vi "Tx to UDP.vi"(7 "Data Conversion":T1, 8 "error in (no error)":errorcluster, 10 "Tx Array":dbl[](array[numeric]), 11 "Header Info":bool[](array[boolean])) -> (0 "error out":errorcluster, 2 "Tx String":string, 5 "Data Conversion out":T1)   [LabVIEW 2016, in "UDP-Custom-Device Engine.lvlib"]
uses:
  UDP-Custom-Device Engine.lvlib
  Types/Engine - Data Conversion Config.ctl
  <vilib>/NI Veristand/VeriStand Data/Library/Byte Buffer/Byte Buffer.lvclass
  <vilib>/NI Veristand/VeriStand Data/Library/Byte Buffer/Byte Buffer.Mapping.ctl
  <vilib>/NI Veristand/VeriStand Data/Library/Typedefs/Typedefs.Data Types.ctl
  <vilib>/NI Veristand/VeriStand Data/Library/Byte Buffer/Byte Buffer.lvclass/Byte Buffer.ctl
  <vilib>/NI Veristand/VeriStand Data/Library/Pointer Operations/Pointer.Write (DBL).vi
  <vilib>/NI Veristand/VeriStand Data/Library/Memory Management/Memory Management.MoveDblBlock.Write (Double).vi
  <vilib>/NI Veristand/VeriStand Data/Library/Byte Buffer/Byte Buffer.Write.Typed Array.vi
  <vilib>/NI Veristand/VeriStand Data/Library/Utilities/Utilities.Buffer.Double.vi
  <vilib>/NI Veristand/VeriStand Data/Library/Byte Buffer/Byte Buffer.Write.vi
  <vilib>/NI Veristand/VeriStand Data/Library/Byte Buffer/Byte Buffer.Write (1D Boolean).vi
  <vilib>/NI Veristand/VeriStand Data/Library/Type Conversion/Type Conversion.From Double.Subset.vi
  <vilib>/NI Veristand/VeriStand Data/Library/Type Conversion/Type Conversion.From Double.Subset (1D Boolean).vi
  <vilib>/NI Veristand/VeriStand Data/Library/Byte Buffer/Byte Buffer.Write (1D SGL).vi
  <vilib>/NI Veristand/VeriStand Data/Library/Type Conversion/Type Conversion.From Double.Subset (1D SGL).vi
  <vilib>/NI Veristand/VeriStand Data/Library/Byte Buffer/Byte Buffer.Write (1D DBL).vi
  <vilib>/NI Veristand/VeriStand Data/Library/Byte Buffer/Byte Buffer.Write (1D I8).vi
  <vilib>/NI Veristand/VeriStand Data/Library/Type Conversion/Type Conversion.From Double.Subset (1D I8).vi
  <vilib>/NI Veristand/VeriStand Data/Library/Byte Buffer/Byte Buffer.Write (1D I16).vi
  <vilib>/NI Veristand/VeriStand Data/Library/Type Conversion/Type Conversion.From Double.Subset (1D I16).vi
  <vilib>/NI Veristand/VeriStand Data/Library/Byte Buffer/Byte Buffer.Write (1D I32).vi
  <vilib>/NI Veristand/VeriStand Data/Library/Type Conversion/Type Conversion.From Double.Subset (1D I32).vi
  <vilib>/NI Veristand/VeriStand Data/Library/Byte Buffer/Byte Buffer.Write (1D I64).vi
  <vilib>/NI Veristand/VeriStand Data/Library/Type Conversion/Type Conversion.From Double.Subset (1D I64).vi
  <vilib>/NI Veristand/VeriStand Data/Library/Byte Buffer/Byte Buffer.Write (1D U8).vi
  <vilib>/NI Veristand/VeriStand Data/Library/Type Conversion/Type Conversion.From Double.Subset (1D U8).vi
  <vilib>/NI Veristand/VeriStand Data/Library/Byte Buffer/Byte Buffer.Write (1D U16).vi
  <vilib>/NI Veristand/VeriStand Data/Library/Type Conversion/Type Conversion.From Double.Subset (1D U16).vi
  <vilib>/NI Veristand/VeriStand Data/Library/Byte Buffer/Byte Buffer.Write (1D U32).vi
  <vilib>/NI Veristand/VeriStand Data/Library/Type Conversion/Type Conversion.From Double.Subset (1D U32).vi
  <vilib>/NI Veristand/VeriStand Data/Library/Byte Buffer/Byte Buffer.Write (1D U64).vi
  <vilib>/NI Veristand/VeriStand Data/Library/Type Conversion/Type Conversion.From Double.Subset (1D U64).vi
  <vilib>/NI Veristand/VeriStand Data/Library/Utilities/Utilities.Sizeof.Array.vi
  <vilib>/NI Veristand/VeriStand Data/Library/Type Conversion/Type Conversion.From Double.vi
  <vilib>/NI Veristand/VeriStand Data/Library/Type Conversion/Type Conversion.From Double (1D Boolean).vi
  <vilib>/NI Veristand/VeriStand Data/Library/Type Conversion/Type Conversion.From Double (1D SGL).vi
  <vilib>/NI Veristand/VeriStand Data/Library/Type Conversion/Type Conversion.From Double (1D I8).vi
  <vilib>/NI Veristand/VeriStand Data/Library/Type Conversion/Type Conversion.From Double (1D I16).vi
  <vilib>/NI Veristand/VeriStand Data/Library/Type Conversion/Type Conversion.From Double (1D I32).vi
  <vilib>/NI Veristand/VeriStand Data/Library/Type Conversion/Type Conversion.From Double (1D I64).vi
  <vilib>/NI Veristand/VeriStand Data/Library/Type Conversion/Type Conversion.From Double (1D U8).vi
  <vilib>/NI Veristand/VeriStand Data/Library/Type Conversion/Type Conversion.From Double (1D U16).vi
  <vilib>/NI Veristand/VeriStand Data/Library/Type Conversion/Type Conversion.From Double (1D U32).vi
  <vilib>/NI Veristand/VeriStand Data/Library/Type Conversion/Type Conversion.From Double (1D U64).vi
  <vilib>/NI Veristand/VeriStand Data/Library/Utilities/Utilities.Sizeof.Scalar.vi
  <vilib>/NI Veristand/VeriStand Data/Library/Memory Management/Memory Management.Handle Return.vi
  <vilib>/NI Veristand/VeriStand Data/Library/VeriStand Data.lvlib
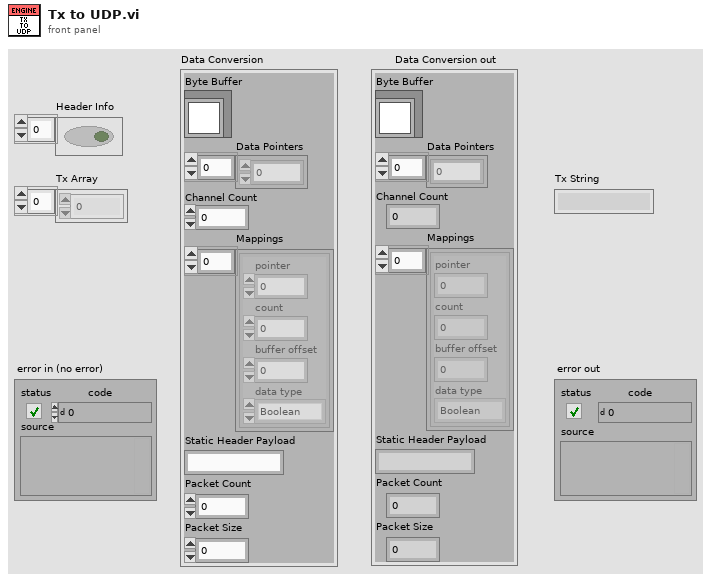
[diagram p1: front panel]
types:
  T1 = typedef "UDP-Custom-Device Engine.lvlib/Engine - Data Conversion Config.ctl" = cluster{"Byte Buffer":refnum<class "Byte Buffer.lvclass">, "Data Pointers":u64[], "Channel Count":i32, "Mappings":T2[], "Static Header Payload":string, "Packet Count":dbl, "Packet Size":i32}
  T2 = typedef "VeriStand Data.lvlib/Byte Buffer.lvclass/Byte Buffer.Mapping.ctl" = cluster{"pointer":u64, "count":i32, "buffer offset":i32, "data type":T3}
  T3 = typedef "VeriStand Data.lvlib/Typedefs.Data Types.ctl" = enum16{"Boolean", "Single", "Double", "I8", "I16", "I32", "I64", "U8", "U16", "U32", "U64"}
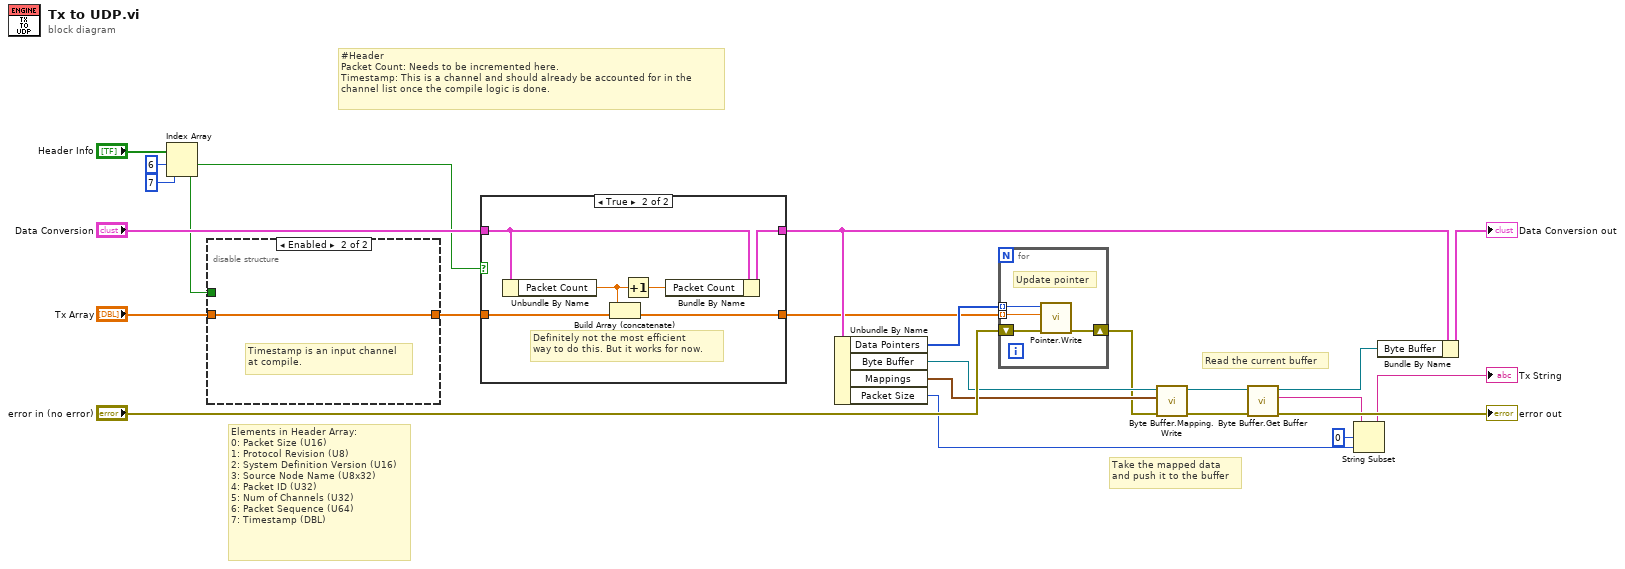
[diagram p0: block diagram]
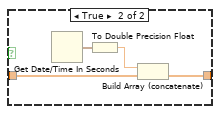
[diagram p3: hidden frame]
diagram:
  # "Elements in Header Array:\n0: Packet Size (U16)\n1: Protocol Revision (U8)\n2: System Definition Version (U16)\n3: Source Node Name (U8x32)\n4: Packet ID (U32)\n5: Num of Channels (U32)\n6: Packet Sequence (U64)\n7: Timestamp (DBL)"
  # "Read the current buffer"
  # "Take the mapped data\nand push it to the buffer"
  # "#Header\nPacket Count: Needs to be incremented here.\nTimestamp: This is a channel and should already be accounted for in the\nchannel list once the compile logic is done."
  n1 = Index Array(array="Header Info", index #1=6 ("index"), index #2=7 ("index")) -> (element #1=w10:bool, element #2=w9:bool)
  n2 = disable-structure shown="Enabled" {
    disable-tunnel: w9 -> [w27 _]
    disable-tunnel: "Tx Array" -> [w26 w33]
    disable-tunnel: [w25 w33] -> w7
    frame Disabled {
      # "#Temp\nThe Timestamp is just set here for now."
      n3 = case shown="False" w27 {
        tunnel: [w28 w31] -> w25
        tunnel: w26 -> [w28 w32]
        frame False {
        }
        frame True {
          n4 = Get Date/Time In Seconds() -> (seconds since 1Jan1904=w30:timestamp)
          n5 = To Double Precision Float(number=w30) -> (double precision float=w29:dbl)
          n6 = Build Array (concatenate)(w29, w32) -> (w31:dbl[])
        }
      }
    }
    frame Enabled {
      # "Timestamp is an input channel\nat compile."
    }
  }
  n7 = case shown="True" w10 {
    tunnel: "Data Conversion" -> [w35 w41]
    tunnel: [w35 w40] -> w13
    tunnel: [w34 w36] -> w5
    tunnel: w7 -> [w34 w37]
    frame False {
    }
    frame True {
      # "Definitely not the most efficient\nway to do this. But it works for now."
      n8 = Unbundle By Name(w41) -> ("Packet Count"=w38:dbl)
      n9 = Build Array (concatenate)(w38, w37) -> (w36:dbl[])
      n10 = Increment(x=w38) -> (x+1=w39:dbl)
      n11 = Bundle By Name(cluster=w41, "Packet Count"=w39) -> (w40:T1)
    }
  }
  n12 = Unbundle By Name(w13) -> ("Data Pointers"=w21:u64[], "Byte Buffer"=w19:refnum<class "Byte Buffer.lvclass">, "Mappings"=w20:T2[], "Packet Size"=w2:i32)
  n13 = for {
    tunnel: w21 -> [w44] mode=indexing
    tunnel: w5 -> [w42] mode=indexing
    shift-right: [w43] -> w18
    shift-left: "error in (no error)" -> [w45]
    # "Update pointer"
    n14 = call-poly <vilib>:"Pointer.Write.vi"("error in (no error)"=w45, "value"=w42, "pointer in"=w44) -> ("error out"=w43:errorcluster)  [unwired: 6 in, 2 out]
  }
  n15 = call <vilib>:"Byte Buffer.Mapping.Write.vi"("error in (no error)"=w18, "mappings"=w20, "Byte Buffer in"=w19) -> ("error out"=w16:errorcluster, "Byte Buffer out"=w17:refnum<class "Byte Buffer.lvclass">)  [unwired: 6 in, 1 out]
  n16 = call <vilib>:"Byte Buffer.Get Buffer.vi"("error in (no error)"=w16, "Byte Buffer in"=w17) -> ("error out"=→"error out":errorcluster, "buffer"=w4:string, "Byte Buffer out"=w15:refnum<class "Byte Buffer.lvclass">)  [unwired: 7 in]
  n17 = String Subset(string=w4, offset (0)=0, length (rest)=w2) -> (substring=→"Tx String":string)
  n18 = Bundle By Name(cluster=w13, "Byte Buffer"=w15) -> (→"Data Conversion out":T1)
